vi "_emi_Loop Control array.vi"(0 "Loop array in":u16[](array[numeric]), 7 "Enable":bool, 11 "error in (no error)":errorcluster) -> (4 "Loop Arrau out":u16[](array[numeric]), 15 "error out":errorcluster)   [LabVIEW 2011]
uses:
  _emi_Loop control int action.ctl
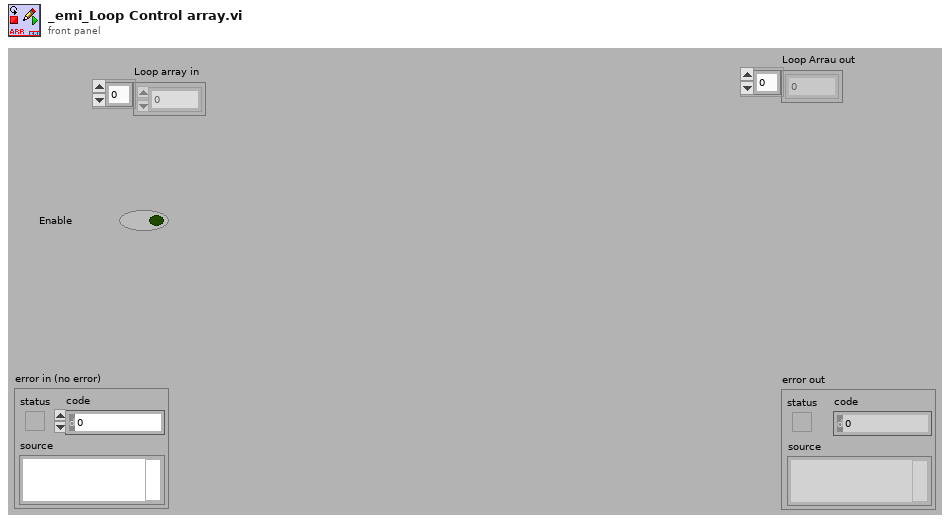
[diagram p1: front panel]
types:
  T1 = typedef "_emi_Loop control int action.ctl" = enum16{"Init index", "Get index", "Set index", "Get Size"}
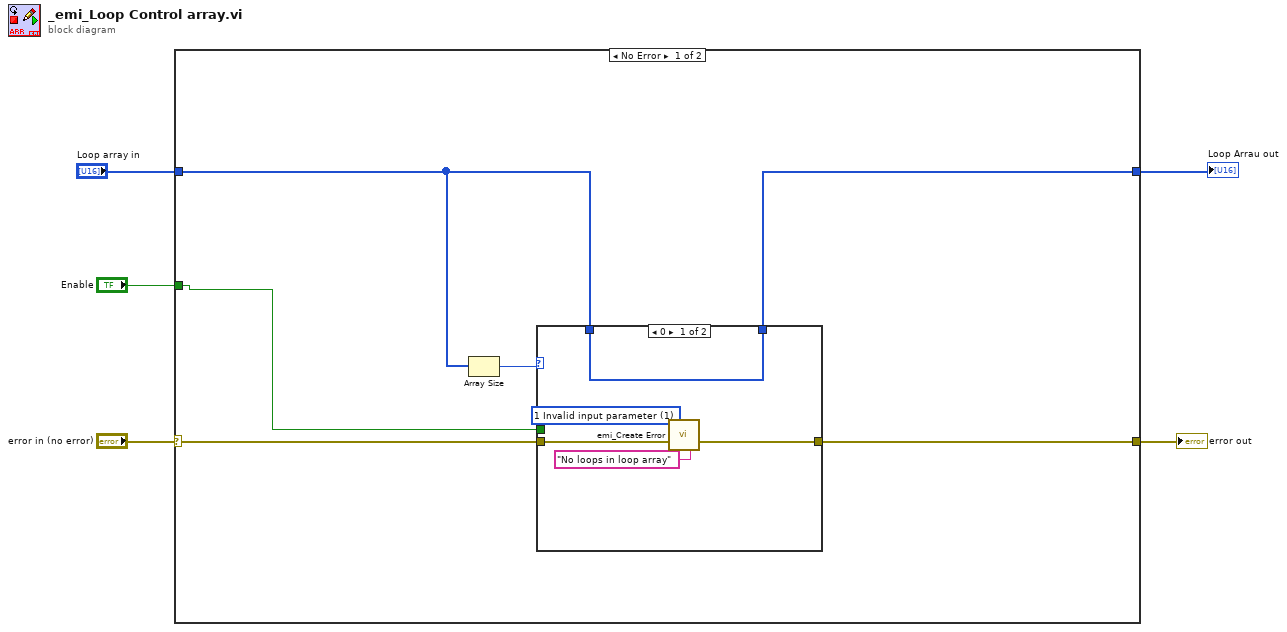
[diagram p0: block diagram]
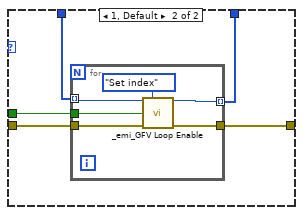
[diagram p2: hidden frame]
diagram:
  n1 = case shown="No Error" "error in (no error)" {
    selector: "error in (no error)" -> [w11 w29]
    tunnel: [w10 w29] -> w4
    tunnel: [w9 w28] -> w1
    tunnel: "Loop array in" -> [w7 w28]
    tunnel: "Enable" -> [w8 _]
    frame No Error {
      n2 = Array Size(array=w7) -> (size(s)=w6:i32)
      n3 = case shown="0" w6 {
        tunnel: w11 -> [w15 w21]
        tunnel: [w14 w20] -> w10
        tunnel: [w16 w19] -> w9
        tunnel: w8 -> [_ w18]
        tunnel: w7 -> [w16 w17]
        frame 0 {
          w13 = 1 items=["0 No Error"=0, "1 Invalid input parameter"=1, "6 Generic file IO "=6, "7 File not Found"=7, "35 Generic Pring Error"=35, "37 Device not Found"=37, "39 Device Unit Error"=39, "40 Could fot Open Device"=40, "42 Generic Error"=42, "52 Unknown Message"=52, "98 Bad File type"=98, "99 Bad File Version"=99, "100 Bad Data in File"=100, "1018 Unspecefied Error"=1018, "1041 Incorrect Password"=1041, "1043 Feature not in this version"=1043, "1109 Unsuported Data type"=1109, "1444 Did not close sucessfully"=1444] ("Error Code")
          n4 = call "emi_Create Error.vi"("Error Code"=w13, "error in (no error)"=w15, "Append String(\"\")"="No loops in loop array" ("Append String(\"\")")) -> ("error out"=w14:errorcluster)  [unwired: 12 in]
        }
        frame 1, Default {
          n5 = for {
            tunnel: w21 -> [w27]
            tunnel: [w26] -> w20
            tunnel: [w25] -> w19 mode=indexing
            tunnel: w18 -> [w24]
            tunnel: w17 -> [w23] mode=indexing
            n6 = call "_emi_GFV Loop Enable.vi"("Loop Index/Numb"=w23, "Action(Get Index)"=_emi_Loop_control_int_action."Set index", "Loop enable In(T)"=w24, "error in (no error)"=w27) -> ("Index out"=w25:u16, "error out"=w26:errorcluster)  [unwired: 8 in, 2 out]
          }
        }
      }
    }
    frame Error {
    }
  }
  "error out" <- w4
  "Loop Arrau out" <- w1
